vi "LoadCommCfg.vi"(8 "error in (no error)":errorcluster, 10 "section (server name)":string, 11 "Client in":refnum<class "Client.lvclass">) -> (0 "error out":errorcluster, 3 "Client out":refnum<class "Client.lvclass">)   [LabVIEW 2018, in "Client.lvclass"]
uses:
  Client.lvclass
  Client.lvclass/Client.ctl
  <vilib>/Utility/config.llb/Read Key (U32).vi
  <vilib>/Utility/config.llb/Read Key (String).vi
  Comm/Stream/Stream.lvclass
  <vilib>/Utility/config.llb/NI_LVConfig.lvlib
panel:
  out "error commfile2":errorcluster
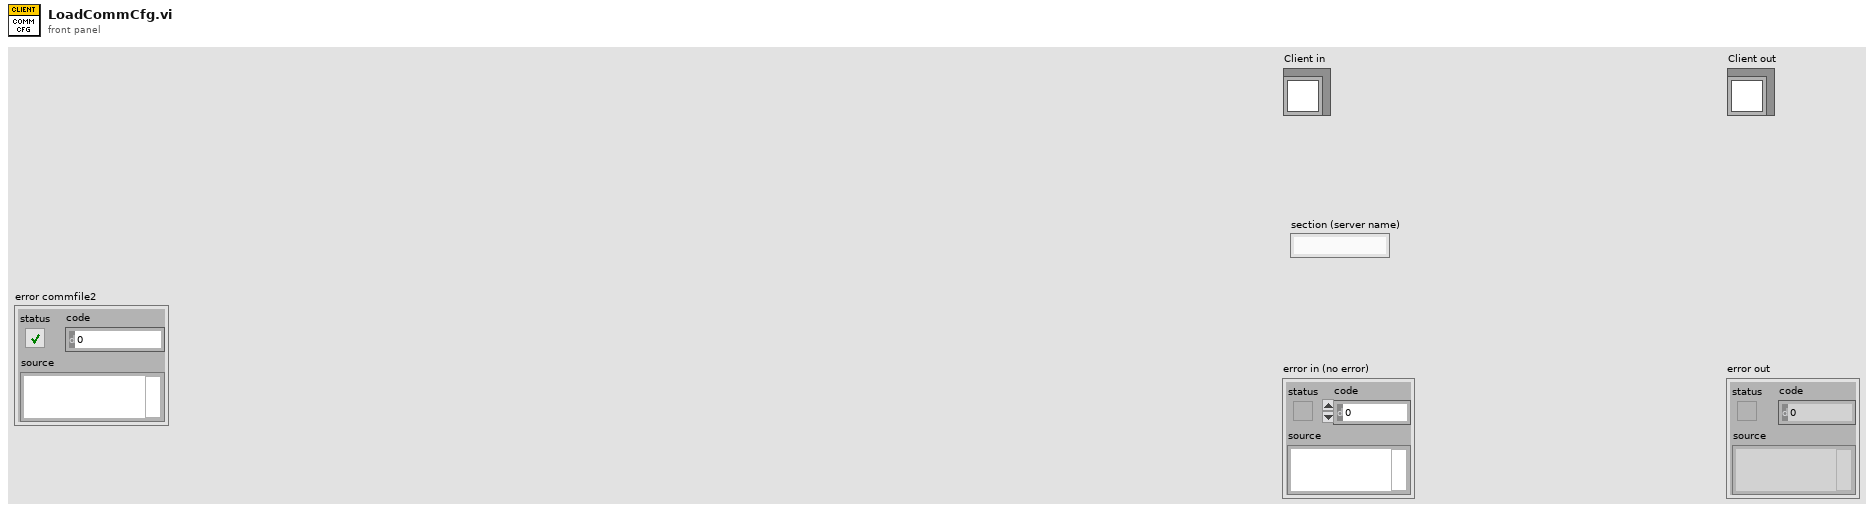
[diagram p1: front panel]
types:
  T1 = typedef "NI_LVConfig.lvlib/Config Data RefNum.ctl" = refnum<k1>
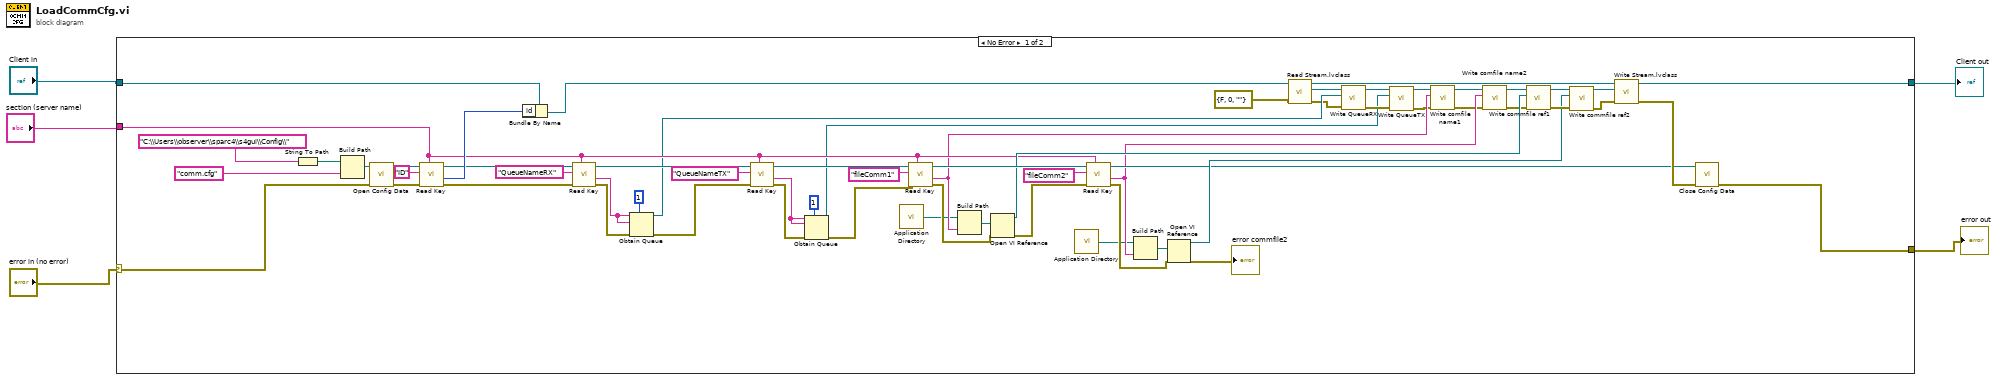
[diagram p0: block diagram]
diagram:
  n1 = case shown="No Error" "error in (no error)" {
    selector: "error in (no error)" -> [w65 w70]
    tunnel: [w62 w70] -> w1
    tunnel: [w50 w69] -> w2
    tunnel: "Client in" -> [w64 w69]
    tunnel: "section (server name)" -> [w33 _]
    frame No Error {
      n2 = String To Path(string="C:\\Users\\observer\\sparc4\\s4gui\\Config\\") -> (path=w6:path)
      n3 = Build Path(base path=w6, name or relative path="comm.cfg") -> (appended path=w11:path)
      n4 = call <vilib>:"Open Config Data.vi"("error in (no error)"=w65, "configuration file path"=w11) -> ("error out"=w66:errorcluster, "refnum"=w68:T1)  [unwired: 7 in, 1 out]
      n5 = call-poly <vilib>:"Read Key.vi"("section"=w33, "error in (no error)"=w66, "key"="ID", "refnum"=w68) -> ("error out"=w53:errorcluster, "value"=w63:u32, "refnum out"=w54:T1)  [unwired: 4 in, 1 out]
      n6 = Bundle By Name(cluster=w64, "id"=w63) -> (w52:refnum<class "Client.lvclass">)
      n7 = call-poly <vilib>:"Read Key.vi"("section"=w33, "error in (no error)"=w53, "key"="QueueNameRX", "refnum"=w54) -> ("error out"=w48:errorcluster, "value"=w60:string, "refnum out"=w59:T1)  [unwired: 4 in, 1 out]
      n8 = Obtain Queue(max queue size (-1, unlimited)=1, name (unnamed)=w60, element data type=w60, error in (no error)=w48) -> (queue out=w20:refnum<queue>, error out=w47:errorcluster)  [unwired: 1 in, 1 out]
      n9 = call-poly <vilib>:"Read Key.vi"("section"=w33, "error in (no error)"=w47, "key"="QueueNameTX", "refnum"=w59) -> ("error out"=w46:errorcluster, "value"=w61:string, "refnum out"=w22:T1)  [unwired: 4 in, 1 out]
      n10 = Obtain Queue(max queue size (-1, unlimited)=1, name (unnamed)=w61, element data type=w61, error in (no error)=w46) -> (queue out=w14:refnum<queue>, error out=w37:errorcluster)  [unwired: 1 in, 1 out]
      n11 = call <vilib>:"Application Directory.vi"() -> ("Application Directory"=w9:path)
      n12 = call-poly <vilib>:"Read Key.vi"("section"=w33, "error in (no error)"=w37, "key"="fileComm1", "refnum"=w22) -> ("error out"=w36:errorcluster, "value"=w28:string, "refnum out"=w45:T1)  [unwired: 4 in, 1 out]
      n13 = Build Path(base path=w9, name or relative path=w28) -> (appended path=w38:path)
      n14 = Open VI Reference(vi path=w38, error in (no error)=w36) -> (vi reference=w34:refnum<vi>, error out=w35:errorcluster)  [unwired: 4 in]
      n15 = call <vilib>:"Application Directory.vi"() -> ("Application Directory"=w8:path)
      n16 = call-poly <vilib>:"Read Key.vi"("section"=w33, "error in (no error)"=w35, "key"="fileComm2", "refnum"=w45) -> ("error out"=w31:errorcluster, "value"=w27:string, "refnum out"=w29:T1)  [unwired: 4 in, 1 out]
      n17 = Build Path(base path=w8, name or relative path=w27) -> (appended path=w32:path)
      n18 = Open VI Reference(vi path=w32, error in (no error)=w31) -> (vi reference=w30:refnum<vi>, error out=→"error commfile2":errorcluster)  [unwired: 4 in]
      n19 = call-dynamic "Read Stream.lvclass.vi"("error in (no error)"=errorcluster {"status"=FALSE, "code"=0, "source"=""}, "Client in"=w52) -> ("error out"=w19:errorcluster, "Stream.lvclass"=w21:refnum<class "Stream.lvclass">, "Client out"=w51:refnum<class "Client.lvclass">)  [unwired: 7 in]
      n20 = call-dynamic "Write QueueRX.vi"("error in (no error)"=w19, "queue RX"=w20, "Stream in"=w21) -> ("error out"=w17:errorcluster, "Stream out"=w18:refnum<class "Stream.lvclass">)  [unwired: 7 in]
      n21 = call-dynamic "Write QueueTX.vi"("error in (no error)"=w17, "queue TX"=w14, "Stream in"=w18) -> ("error out"=w15:errorcluster, "Stream out"=w16:refnum<class "Stream.lvclass">)  [unwired: 7 in]
      n22 = call-dynamic "Write comfile name1.vi"("error in (no error)"=w15, "comfile name1"=w28, "Stream in"=w16) -> ("error out"=w24:errorcluster, "Stream out"=w26:refnum<class "Stream.lvclass">)  [unwired: 7 in]
      n23 = call-dynamic "Write comfile name2.vi"("error in (no error)"=w24, "comfile name2"=w27, "Stream in"=w26) -> ("error out"=w23:errorcluster, "Stream out"=w25:refnum<class "Stream.lvclass">)  [unwired: 7 in]
      n24 = call-dynamic "Write commfile ref1.vi"("error in (no error)"=w23, "commfile ref1"=w34, "Stream in"=w25) -> ("error out"=w40:errorcluster, "Stream out"=w42:refnum<class "Stream.lvclass">)  [unwired: 7 in]
      n25 = call-dynamic "Write commfile ref2.vi"("error in (no error)"=w40, "commfile ref2"=w30, "Stream in"=w42) -> ("error out"=w39:errorcluster, "Stream out"=w41:refnum<class "Stream.lvclass">)  [unwired: 7 in]
      n26 = call-dynamic "Write Stream.lvclass.vi"("error in (no error)"=w39, "Stream.lvclass"=w41, "Client in"=w51) -> ("error out"=w49:errorcluster, "Client out"=w50:refnum<class "Client.lvclass">)  [unwired: 7 in]
      n27 = call <vilib>:"Close Config Data.vi"("error in (no error)"=w49, "refnum"=w29) -> ("error out"=w62:errorcluster)  [unwired: 8 in, 1 out]
    }
    frame Error {
    }
  }
  "error out" <- w1
  "Client out" <- w2
